vi "Video Stuff v05.vi"() -> ()   [LabVIEW 2009]
uses:
  <vilib>/userDefined/High Color/IMAQdx.ctl
  <vilib>/vision/NI_Vision_Development_Module.lvlib
  <vilib>/vision/driver/NI_Vision_Acquisition_Software.lvlib
panel:
  out "Occupancy Grid Square Size":dbl
  in  "LIDAR/Wheel Position Offset (in.)":dbl=30.0
  out "\"Obstickles\" y":dbl[](array[numeric])
  out "\"Obstickles\" x":dbl[](array[numeric])
  in  "Max Width of Vision (in.)":i32=84
  out "Small":T1(plugin-control)
  in  "Resolution of Small Image":i32=36
  out "Super Filter":T1(plugin-control)
  in  "Color Mode":u16(ring) items=["RGB", "HSL", "HSV", "HSI"]
  in  "Blue Range":cluster{"Lower value":i32, "Upper value":i32}={"Lower value"=250, "Upper value"=255}
  in  "Green Range":cluster{"Lower value":i32, "Upper value":i32}={"Lower value"=250, "Upper value"=255}
  in  "Red Range":cluster{"Lower value":i32, "Upper value":i32}={"Lower value"=240, "Upper value"=255}
  in  "stop":bool
  out "trans":T1(plugin-control)
  out "Buffer Number":u32
  out "Live Video":T1(plugin-control)
  in  "Video Modes":i32(listbox)
  in  "Camera Name":T2="cam0"
  in  "Calibration File Path":path=path "C:/Documents and Settings/ekolker/My Documents/OGRE/to be synched/calibrationGrid.PNG"
  out "Top Image":T1(plugin-control) caption="Calibration Template"
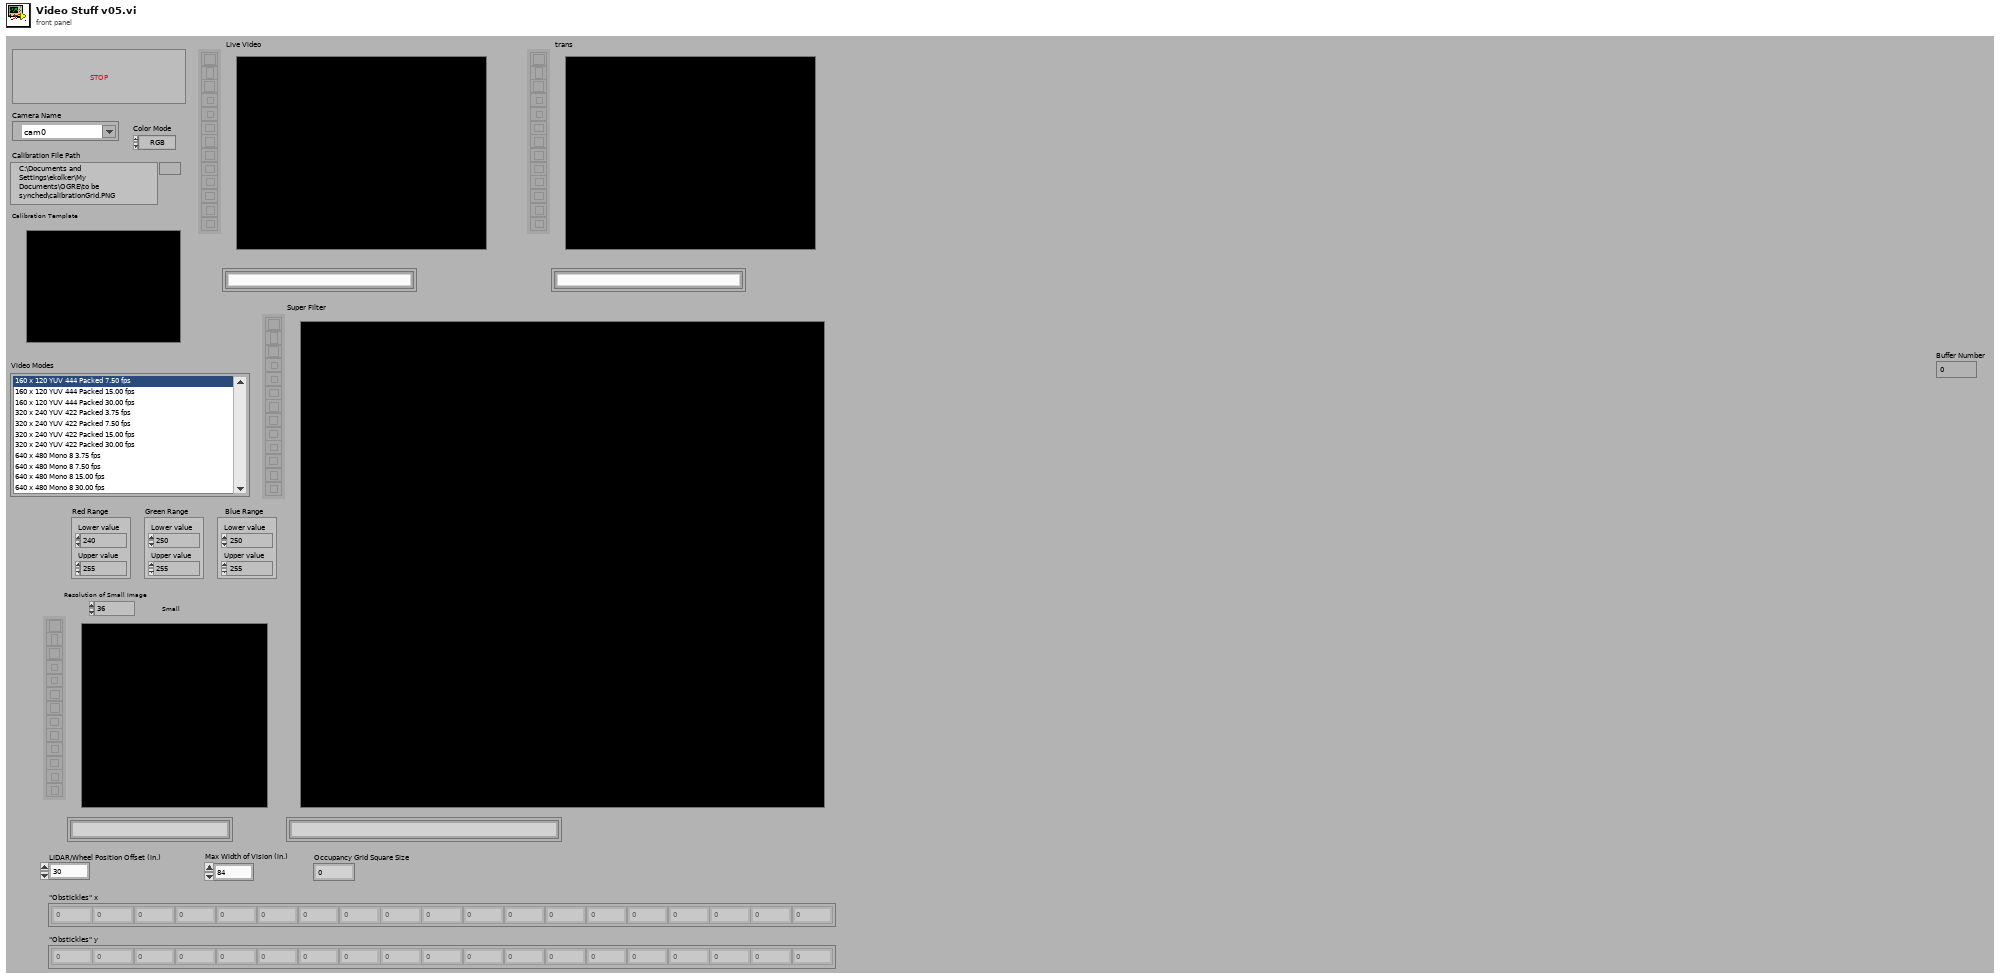
[diagram p1: front panel]
types:
  T1 = typedef "IMAQ Image.ctl" = refnum<image>
  T2 = typedef "IMAQdx.ctl" = refnum<k21>
  T3 = typedef "Image Type" = u32
  T4 = cluster{"X Step":sgl, "Y Step":sgl, "Unit":u32, "Threshold Range":cluster{"Lower value":sgl, "Upper value":sgl}}
  T5 = cluster{"Distortion":u32, "Corrected Image Scaling":u32, "Corrected Image Learn ROI":u32, "Learn Error Map?":bool, "Learn Correction Table?":bool}
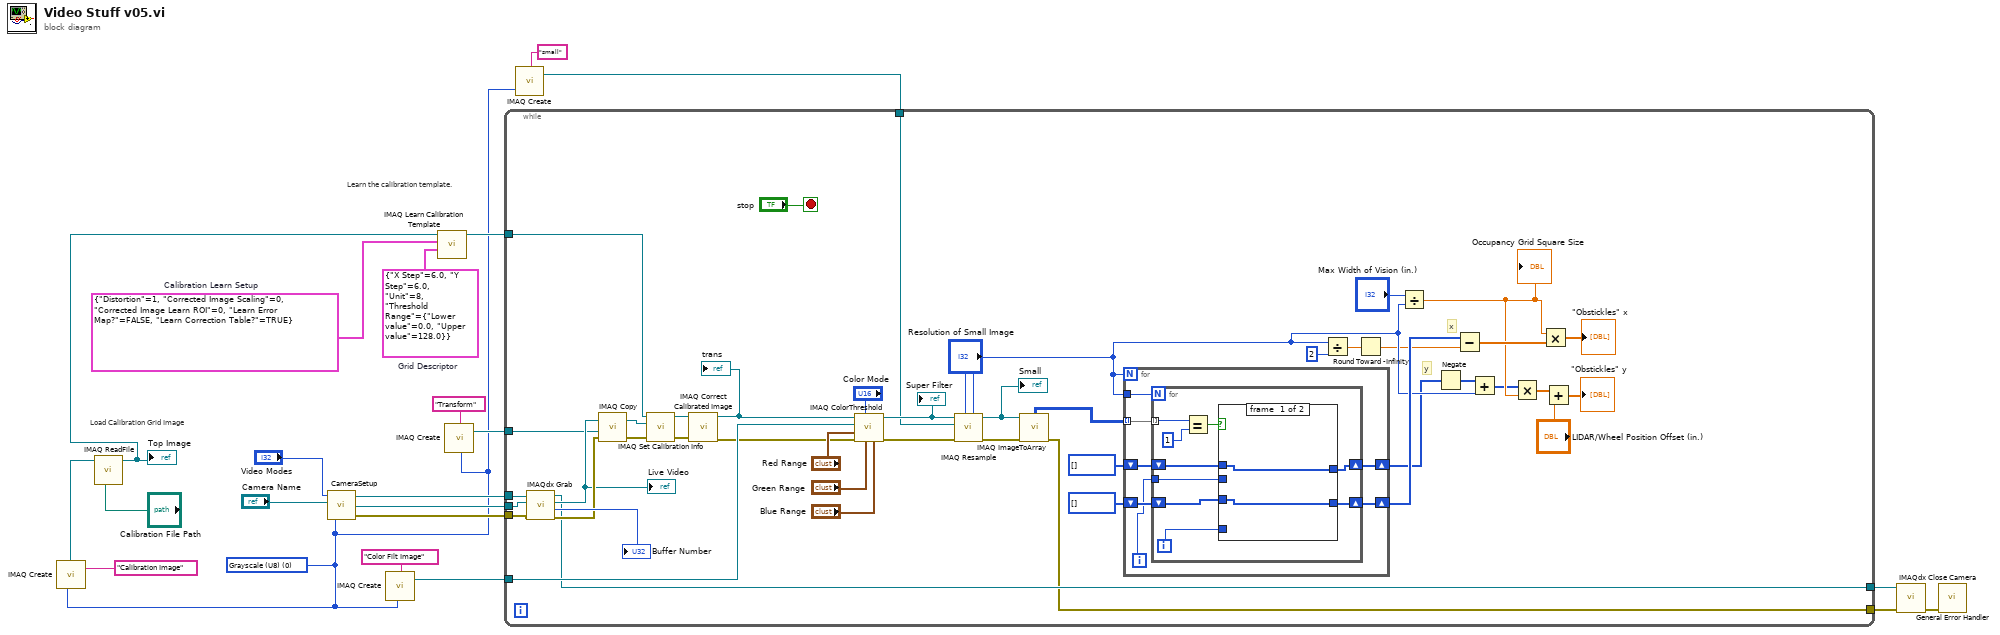
[diagram p0: block diagram]
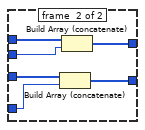
[diagram p2: hidden frame]
diagram:
  w5 = T3 0 items=["Grayscale (U8)", "Grayscale (I16)", "Grayscale (SGL)", "Complex (CSG)", "RGB (U32)", "HSL (U32)", "RGB (U64)", "Grayscale (U16)"] ("Image Type")
  w21 = T4 {"X Step"=6.0, "Y Step"=6.0, "Unit"=8, "Threshold Range"={"Lower value"=0.0, "Upper value"=128.0}}  # Grid Descriptor
  w22 = T5 {"Distortion"=1, "Corrected Image Scaling"=0, "Corrected Image Learn ROI"=0, "Learn Error Map?"=FALSE, "Learn Correction Table?"=TRUE}  # Calibration Learn Setup
  # "Load Calibration Grid Image"
  # "Learn the calibration template."
  n1 = call "IMAQ Create"("Image Name"="Calibration Image", "Image Type"=w5) -> ("New Image"=w9:T1)  [unwired: 2 in, 2 out]
  n2 = call "IMAQ ReadFile"("File Path"="Calibration File Path", "Image"=w9) -> ("Image Out"=w8:T1)  [unwired: 3 in, 6 out]
  "Top Image" <- w8
  n3 = call "CameraSetup.vi"("Image Type"=w5, "Camera Name"="Camera Name", "Video Modes"="Video Modes") -> ("error out"=w10:errorcluster, "New Image"=w11:T1, "Session Out"=w12:T2)  [unwired: 1 in]
  n4 = call "IMAQ Create"("Image Name"="Color Filt Image", "Image Type"=w5) -> ("New Image"=w7:T1)  [unwired: 2 in, 2 out]
  n5 = call "IMAQ Learn Calibration Template"("Grid Descriptor"=w21, "Calibration Learn Setup"=w22, "Image"=w8) -> ("Calibrated Image"=w14:T1)  [unwired: 4 in, 4 out]
  n6 = call "IMAQ Create"("Image Name"="Transform", "Image Type"=w5) -> ("New Image"=w13:T1)  [unwired: 2 in, 2 out]
  n7 = call "IMAQ Create"("Image Name"="small", "Image Type"=w5) -> ("New Image"=w4:T1)  [unwired: 2 in, 2 out]
  n8 = while {
    tunnel: w14 -> [w60]
    tunnel: w13 -> [w59]
    tunnel: w12 -> [w58]
    tunnel: w11 -> [w57]
    tunnel: w10 -> [w56]
    tunnel: w7 -> [w45]
    tunnel: w4 -> [w43]
    tunnel: [w41] -> w2
    tunnel: [w40] -> w1
    stop <- "stop" stop-if-true
    # "y"
    # "x"
    n9 = call <vilib>:"IMAQdx Grab.vi"("error in"=w56, "Image In"=w57, "Session In"=w58) -> ("error out"=w62:errorcluster, "Buffer Number Out"=→"Buffer Number":u32, "Image Out"=w61:T1, "Session Out"=w41:T2)  [unwired: 1 in, 4 out]
    "Live Video" <- w61
    n10 = call "IMAQ Copy"("error in (no error)"=w62, "Image Dst"=w59, "Image Src"=w61) -> ("error out"=w63:errorcluster, "Image Dst Out"=w66:T1)  [unwired: 3 in]
    n11 = call "IMAQ Set Calibration Info"("error in (no error)"=w63, "Image Dst"=w66, "Image Src"=w60) -> ("error out"=w64:errorcluster, "Calibrated Image"=w65:T1)  [unwired: 1 in, 6 out]
    n12 = call "IMAQ Correct Calibrated Image"("error in (no error)"=w64, "Image Src"=w65) -> ("error out"=w44:errorcluster, "Corrected Image"=w46:T1)  [unwired: 5 in, 3 out]
    "trans" <- w46
    n13 = call "IMAQ ColorThreshold"("Blue or Luma or Val or Inten Range"="Blue Range", "Green or Sat Range"="Green Range", "Color Mode"="Color Mode", "error in (no error)"=w44, "Red or Hue Range"="Red Range", "Image Dst"=w45, "Image Src"=w46) -> ("error out"=w51:errorcluster, "Image Dst Out"=w50:T1)  [unwired: 3 in]
    "Super Filter" <- w50
    n14 = call "IMAQ Resample"("X Resolution"="Resolution of Small Image", "Y Resolution"="Resolution of Small Image", "error in (no error)"=w51, "Image Dst"=w43, "Image Src"=w50) -> ("error out"=w49:errorcluster, "Image Dst Out"=w48:T1)  [unwired: 5 in]
    "Small" <- w48
    n15 = call "IMAQ ImageToArray"("error in (no error)"=w49, "Image"=w48) -> ("error out"=w40:errorcluster, "Image Pixels (U8)"=w37:u8[][])  [unwired: 2 in, 3 out]
    n16 = for {
      N: "Resolution of Small Image" -> [_]
      tunnel: "Resolution of Small Image" -> [w74]
      tunnel: w37 -> [w73] mode=indexing
      shift-right: [w72] -> w36
      shift-left: i32[] [] -> [w71]
      shift-right: [w69] -> w25
      shift-left: i32[] [] -> [w68]
      i -> [w70]
      n17 = for {
        N: w74 -> [_]
        tunnel: w73 -> [w83] mode=indexing
        shift-right: [w79] -> w72
        shift-left: w71 -> [w78]
        tunnel: w70 -> [w77]
        shift-right: [w76] -> w69
        shift-left: w68 -> [w75]
        i -> [w81]
        n18 = Equal?(x=w83, y=u8 1) -> (x = y?=w80:bool)
        n19 = case shown="False" w80 {
          tunnel: w81 -> [_ w91]
          tunnel: [w84 w90] -> w79
          tunnel: w78 -> [w84 w89]
          tunnel: w77 -> [_ w88]
          tunnel: [w85 w87] -> w76
          tunnel: w75 -> [w85 w86]
          frame #0 {
          }
          frame #1 {
            n20 = Build Array (concatenate)(w89, w91) -> (w90:i32[])
            n21 = Build Array (concatenate)(w86, w88) -> (w87:i32[])
          }
        }
      }
    }
    n22 = Divide(x="Resolution of Small Image", y=2) -> (x/y=w24:dbl)
    n23 = Round Toward -Infinity(1:w24) -> (0:w23:dbl)
    n24 = Divide(x="Max Width of Vision (in.)", y="Resolution of Small Image") -> (x/y=w31:dbl)
    "Occupancy Grid Square Size" <- w31
    n25 = Negate(x=w25) -> (-x=w26:i32[])
    n26 = Subtract(x=w36, y=w23) -> (x-y=w32:dbl[])
    n27 = Add(x=w26, y="Resolution of Small Image") -> (x+y=w30:i32[])
    n28 = Multiply(x=w30, y=w31) -> (x*y=w27:dbl[])
    n29 = Multiply(x=w31, y=w32) -> (x*y=→"\"Obstickles\" x":dbl[])
    n30 = Add(x=w27, y="LIDAR/Wheel Position Offset (in.)") -> (x+y=→"\"Obstickles\" y":dbl[])
  }
  n31 = call <vilib>:"IMAQdx Close Camera.vi"("error in"=w1, "Session In"=w2) -> ("error out"=w3:errorcluster)  [unwired: 9 out]
  n32 = call <vilib>:"General Error Handler.vi"("error in (no error)"=w3) -> ()  [unwired: 1 in, 14 out]
